vi "Launcher.vi"() -> ()   [LabVIEW 2024]
uses:
  TrafficLight_class/TrafficLight.lvclass
  <vilib>/Utility/miscctls.llb/LVRectTypeDef.ctl
panel:
  out "GREENLIGHT":u32(colorbox)
  out "YELLOWLIGHT":u32(colorbox)
  out "REDLIGHT":u32(colorbox)
  # "Made by Ramazan Burak Korkmaz"
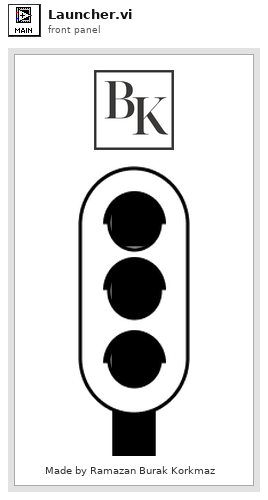
[diagram p1: front panel]
types:
  T1 = typedef "LVRectTypeDef.ctl" = cluster{"Left":i16, "Top":i16, "Right":i16, "Bottom":i16}
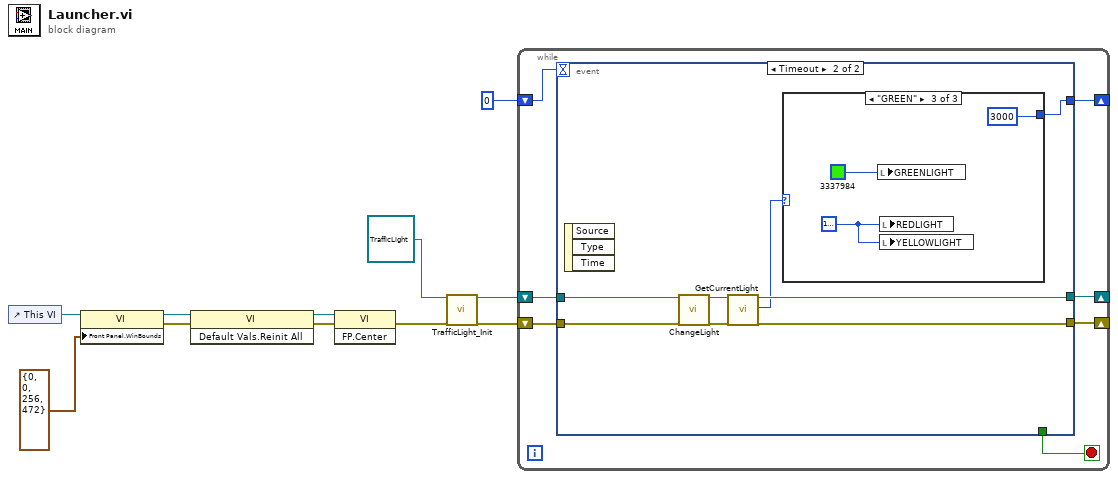
[diagram p0: block diagram]
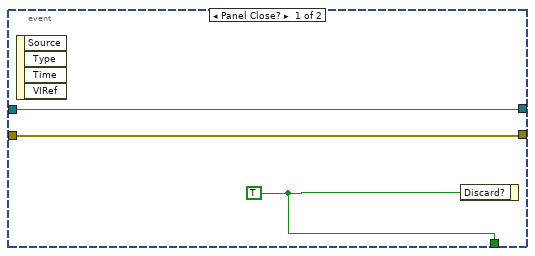
[diagram p2: hidden frame]
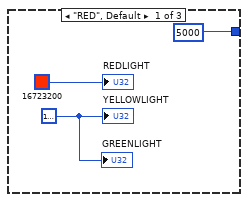
[diagram p3: hidden frame]
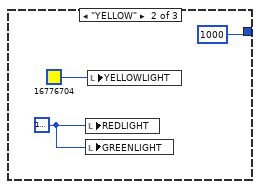
[diagram p4: hidden frame]
diagram:
  n1 = control-ref of="This VI"() -> (w7:refnum<vi>)
  n2 = property class="VI"(reference=w7, "Front Panel.WinBounds"=T1 {"Left"=0, "Top"=0, "Right"=256, "Bottom"=472} ("Front Panel Window:Window Bounds")) -> (reference out=w6:refnum<vi>, error out=w5:errorcluster)  [unwired: 1 in]
  n3 = invoke class="VI" method="Default Vals.Reinit All"(reference=w6, error in=w5) -> (reference out=w4:refnum<vi>, error out=w3:errorcluster)  [unwired: 1 in, 1 out]
  n4 = invoke class="VI" method="FP.Center"(reference=w4, error in=w3) -> (error out=w2:errorcluster)  [unwired: 1 in, 2 out]
  n5 = call "TrafficLight_Init.vi"("object in"=refnum<class "TrafficLight.lvclass"> refnum ("TrafficLight"), "Error In"=w2) -> ("object out"=w10:refnum<class "TrafficLight.lvclass">, "Error Out"=w9:errorcluster)  [unwired: 16 in]
  n6 = while {
    shift-right: [w16] -> _
    shift-left: w10 -> [w18]
    shift-right: [w15] -> _
    shift-left: w9 -> [w17]
    shift-right: [w12] -> _
    shift-left: 0 -> [w13]
    stop <- w14 stop-if-true
    n7 = event shown="[1] Timeout" {
      selector: _ -> [_ _]
      dyn-events: _ -> [_ _]
      timeout: w13 -> [_ _]
      tunnel: w18 -> [w20 w24]
      tunnel: w17 -> [w19 w29]
      tunnel: [w20 w27] -> w16
      tunnel: [w19 w28] -> w15
      tunnel: [w21 _] -> w14
      tunnel: [_ w22] -> w12
      event Panel Close? {
        w21 = TRUE ("Discard?")
        n8 = event-data() -> ()  [unwired: 1 in, 4 out]
        n9 = event-data("Discard?"=w21) -> ()  [unwired: 1 in, 1 out]
      }
      event Timeout {
        n10 = event-data() -> ()  [unwired: 1 in, 3 out]
        n11 = call-dynamic "ChangeLight.vi"("object in"=w24, "Error In"=w29) -> ("object out"=w23:refnum<class "TrafficLight.lvclass">, "Error Out"=w25:errorcluster)  [unwired: 16 in]
        n12 = call-dynamic "GetCurrentLight.vi"("object in"=w23, "Error In"=w25) -> ("object out"=w27:refnum<class "TrafficLight.lvclass">, "CurrentLight"=w26:enum16{"RED", "YELLOW", "GREEN"}, "Error Out"=w28:errorcluster)  [unwired: 15 in]
        n13 = case shown="\"GREEN\"" w26 {
          tunnel: [5000 1000 3000] -> w22
          frame "RED", Default {
            w32 = u32 16777226 ("YELLOWLIGHT")
            "YELLOWLIGHT" <- w32
            "GREENLIGHT" <- w32
            "REDLIGHT" <- u32 16723200 ("REDLIGHT")
          }
          frame "YELLOW" {
            w34 = u32 16777226 ("REDLIGHT")
            n14 = local write "REDLIGHT"(w34) -> ()
            n15 = local write "GREENLIGHT"(w34) -> ()
            n16 = local write "YELLOWLIGHT"(u32 16776704 ("YELLOWLIGHT")) -> ()
          }
          frame "GREEN" {
            w37 = u32 16777226 ("REDLIGHT")
            n17 = local write "GREENLIGHT"(u32 3337984 ("GREENLIGHT")) -> ()
            n18 = local write "REDLIGHT"(w37) -> ()
            n19 = local write "YELLOWLIGHT"(w37) -> ()
          }
        }
      }
    }
  }
